vi "rs3 wait for frames4.vi"(8 "error in (no error)":errorcluster, 11 "device in":u64) -> (0 "error out":errorcluster, 3 "device out":u64)   [LabVIEW 2017, in "libRealSense3.lvlib"]
doc: "Block until new frames are available. Returns the next FRAME handle when available."
uses:
  <vilib>/addons/RealSense/libRealSense3.lvlib
  <vilib>/addons/RealSense/realsense-d.dll
panel:
  # "RS3 Wait for Frames"
  # "(C) Intel Corp. 2017,  AGJ"
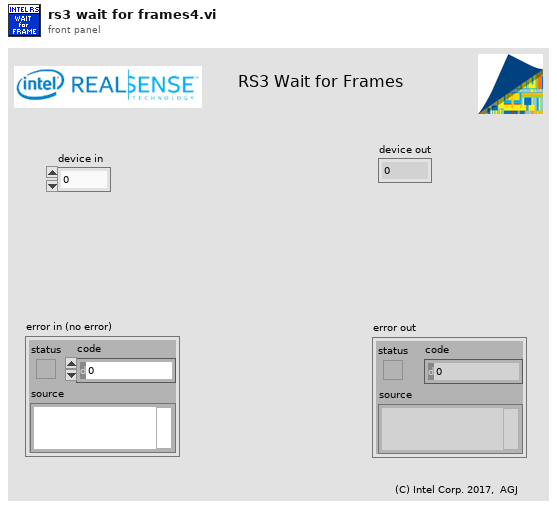
[diagram p1: front panel]
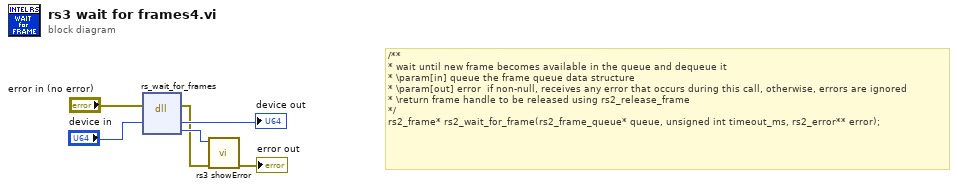
[diagram p0: block diagram]
diagram:
  # "/**\n* wait until new frame becomes available in the queue and dequeue it\n* \\param[in] queue the frame queue data structure\n* \\param[out] error  if non-null, receives any error that occurs during this call, otherwise, errors are ignored\n* \\return frame handle to be released using rs2_release_frame\n*/\nrs2_frame* rs2_wait_for_frame(rs2_frame_queue* queue, unsigned int timeout_ms, rs2_error** error);"
  n1 = dll-call lib="C:/Program Files (x86)/National Instruments/LabVIEW 2017/vi.lib/addons/RealSense/realsense-d.dll" fn="rs_wait_for_frames"(error in="error in (no error)", "device"="device in") -> (error out=w2:errorcluster, "device"=→"device out":u64, "error"=w3:u64)  [unwired: 4 in, 1 out]
  n2 = call <vilib>:"rs3 showError.vi"("error in (no error)"=w2, "error"=w3) -> ("error out"=→"error out":errorcluster)  [unwired: 5 in, 4 out]
